vi "Keithley 6220_1 set current.vi"(7 "Change output":bool=TRUE, 8 "error in (no error)":errorcluster, 9 "Current (A)":dbl=0.001 min=-1050.0 max=1050.0 step=1.0 format="%.4p", 10 "Output ON":bool, 11 "VISA resource name":refnum<visa-resource-name>) -> (0 "error out":errorcluster, 3 "VISA resource name out":refnum<visa-resource-name>)   [LabVIEW 2015]
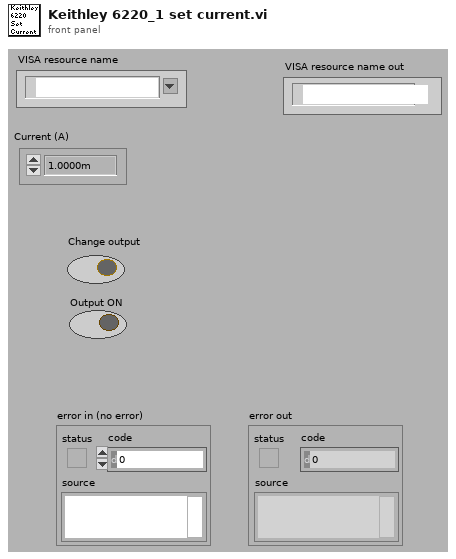
[diagram p1: front panel]
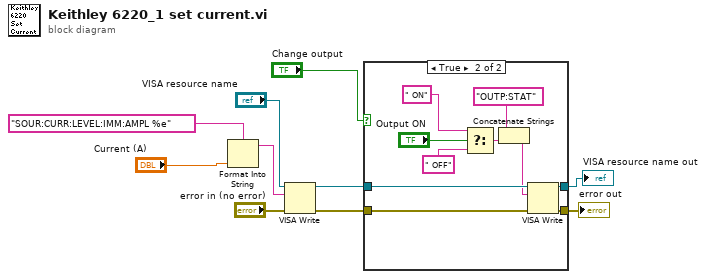
[diagram p0: block diagram]
diagram:
  n1 = Format Into String(format string="SOUR:CURR:LEVEL:IMM:AMPL %e", "Current (A)") -> (resulting string=w6:string)  [unwired: 2 in, 1 out]
  n2 = VISA Write(VISA resource name="VISA resource name", write buffer=w6, error in (no error)="error in (no error)") -> (VISA resource name out=w5:refnum<visa-resource-name>, error out=w3:errorcluster)  [unwired: 1 out]
  n3 = case shown="True" "Change output" {
    tunnel: w5 -> [w12 w22]
    tunnel: [w12 w21] -> w4
    tunnel: w3 -> [w11 w19]
    tunnel: [w11 w18] -> w2
    frame False {
    }
    frame True {
      n4 = Select(t=" ON", s="Output ON", f=" OFF") -> (s? t:f=w13:string)
      n5 = Concatenate Strings("OUTP:STAT", w13) -> (w14:string)
      n6 = VISA Write(VISA resource name=w22, write buffer=w14, error in (no error)=w19) -> (VISA resource name out=w21:refnum<visa-resource-name>, error out=w18:errorcluster)  [unwired: 1 out]
    }
  }
  "VISA resource name out" <- w4
  "error out" <- w2
